vi "HW_GEN - Construct Modu Tag.vi"(7 "ChanType":string, 10 "ModSN":string, 11 "ModName":string) -> (3 "String":string)   [LabVIEW 2016]
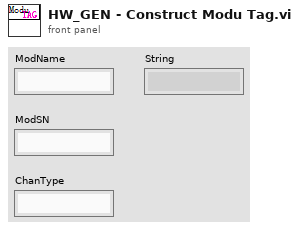
[diagram p1: front panel]
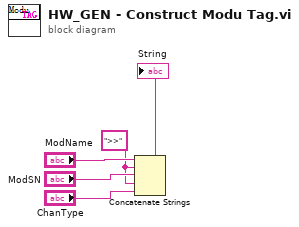
[diagram p0: block diagram]
diagram:
  w1 = ">>" ("string")
  n1 = Concatenate Strings("ModName", w1, "ModSN", w1, "ChanType") -> (→"String":string)
